vi "仪器控制1.vi"() -> ()   [LabVIEW 2018]
uses:
  <vilib>/Instr/_visa.llb/VISA Configure Serial Port (Instr).vi
panel:
  in  "截取采样时间下限":dbl
  in  "截取采样时间上限":dbl
  out "已循环周期数":i32
  in  "停止":bool
  out "x-y":u32
  out "停止按钮指示灯 2":bool
  out "大小":i32
  out "原始数据":dbl
  in  "偏差范围上限 2":dbl=5.0
  in  "偏差范围下限 2":dbl=5.0
  out "电流超出范围":bool=TRUE
  out "电流上限":dbl
  out "电流下限":dbl
  in  "截取下限时间 2":dbl
  in  "截取上限时间 2":dbl
  in  "截取下限时间":dbl=1.0
  in  "截取上限时间":dbl=10.0
  out "当前时间值":dbl
  out "波形图（采样频率不够无法完全拟合出曲线c）":dbl[](graph)
  out "子字符串之前 2":string
  out "双精度浮点数":dbl
  out "*(类型 *) &x":dbl
  out "实际输出电流":dbl
  out "子字符串之后":string
  out "匹配子字符串":string
  out "子字符串之前":string
  out "读取缓冲区":string
  out "运行按钮指示灯":bool
  in  "退出":bool
  in  "运行":bool
  in  "前段波形持续时间(s)":dbl=10.0
  in  "斜率决定因素":dbl=0.02
  in  "循环周期数":i32=30000
  out "第一周期近似波形图":dbl[](graph)
  in  "0安培电流保持时间":dbl=50.0
  in  "Time Resolution(s)":dbl=0.025
  in  "IR":dbl=20.0
  # "截取采样时间上限与斜率决定因素保持一致"
  # "配置"
  # "初始电流：50A 斜率决定因素：0.05\n初始电流：20A 斜率决定因素：0.02\n斜率决定因素值越小，越倾斜，但有过冲的风险越大\n总结：初始电流越大，斜率决定因素应越大"
  # "检测"
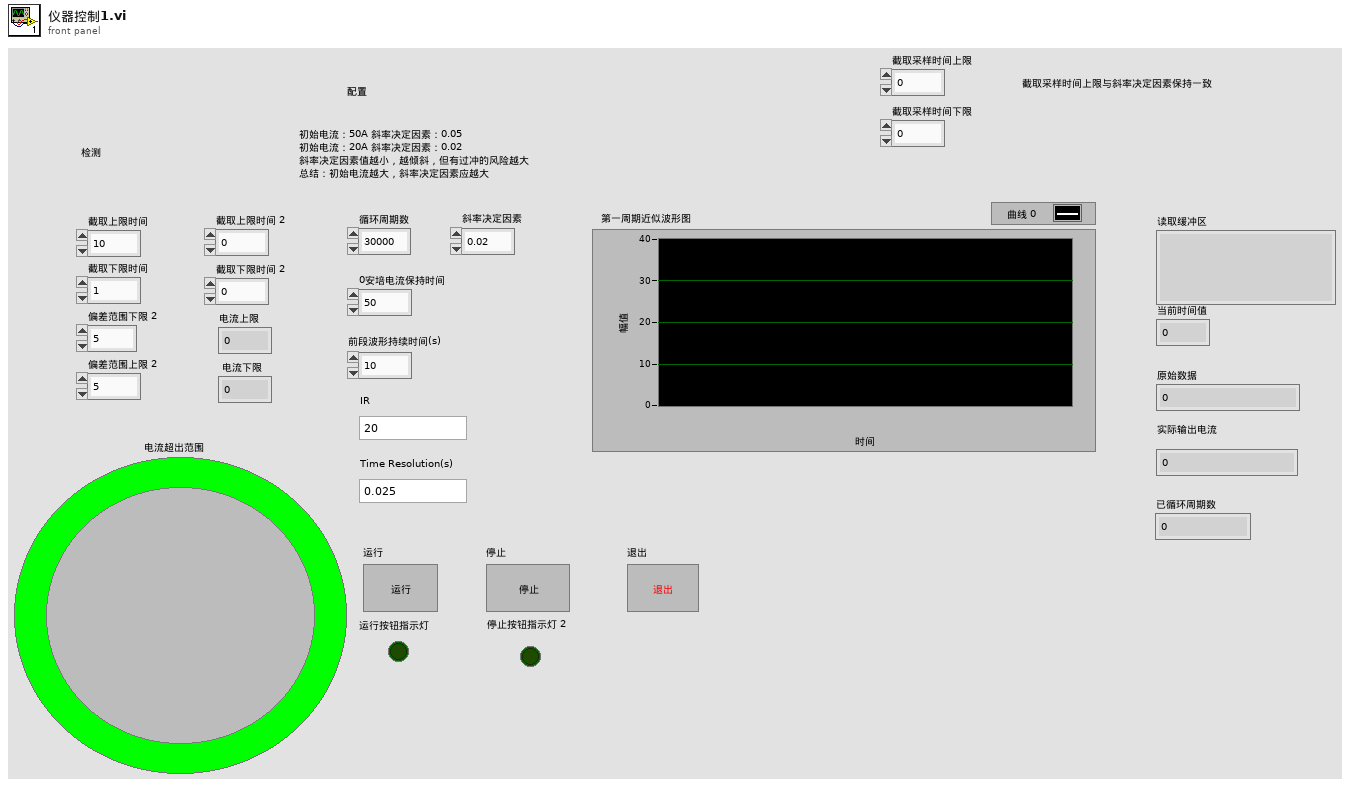
[diagram p1: front panel]
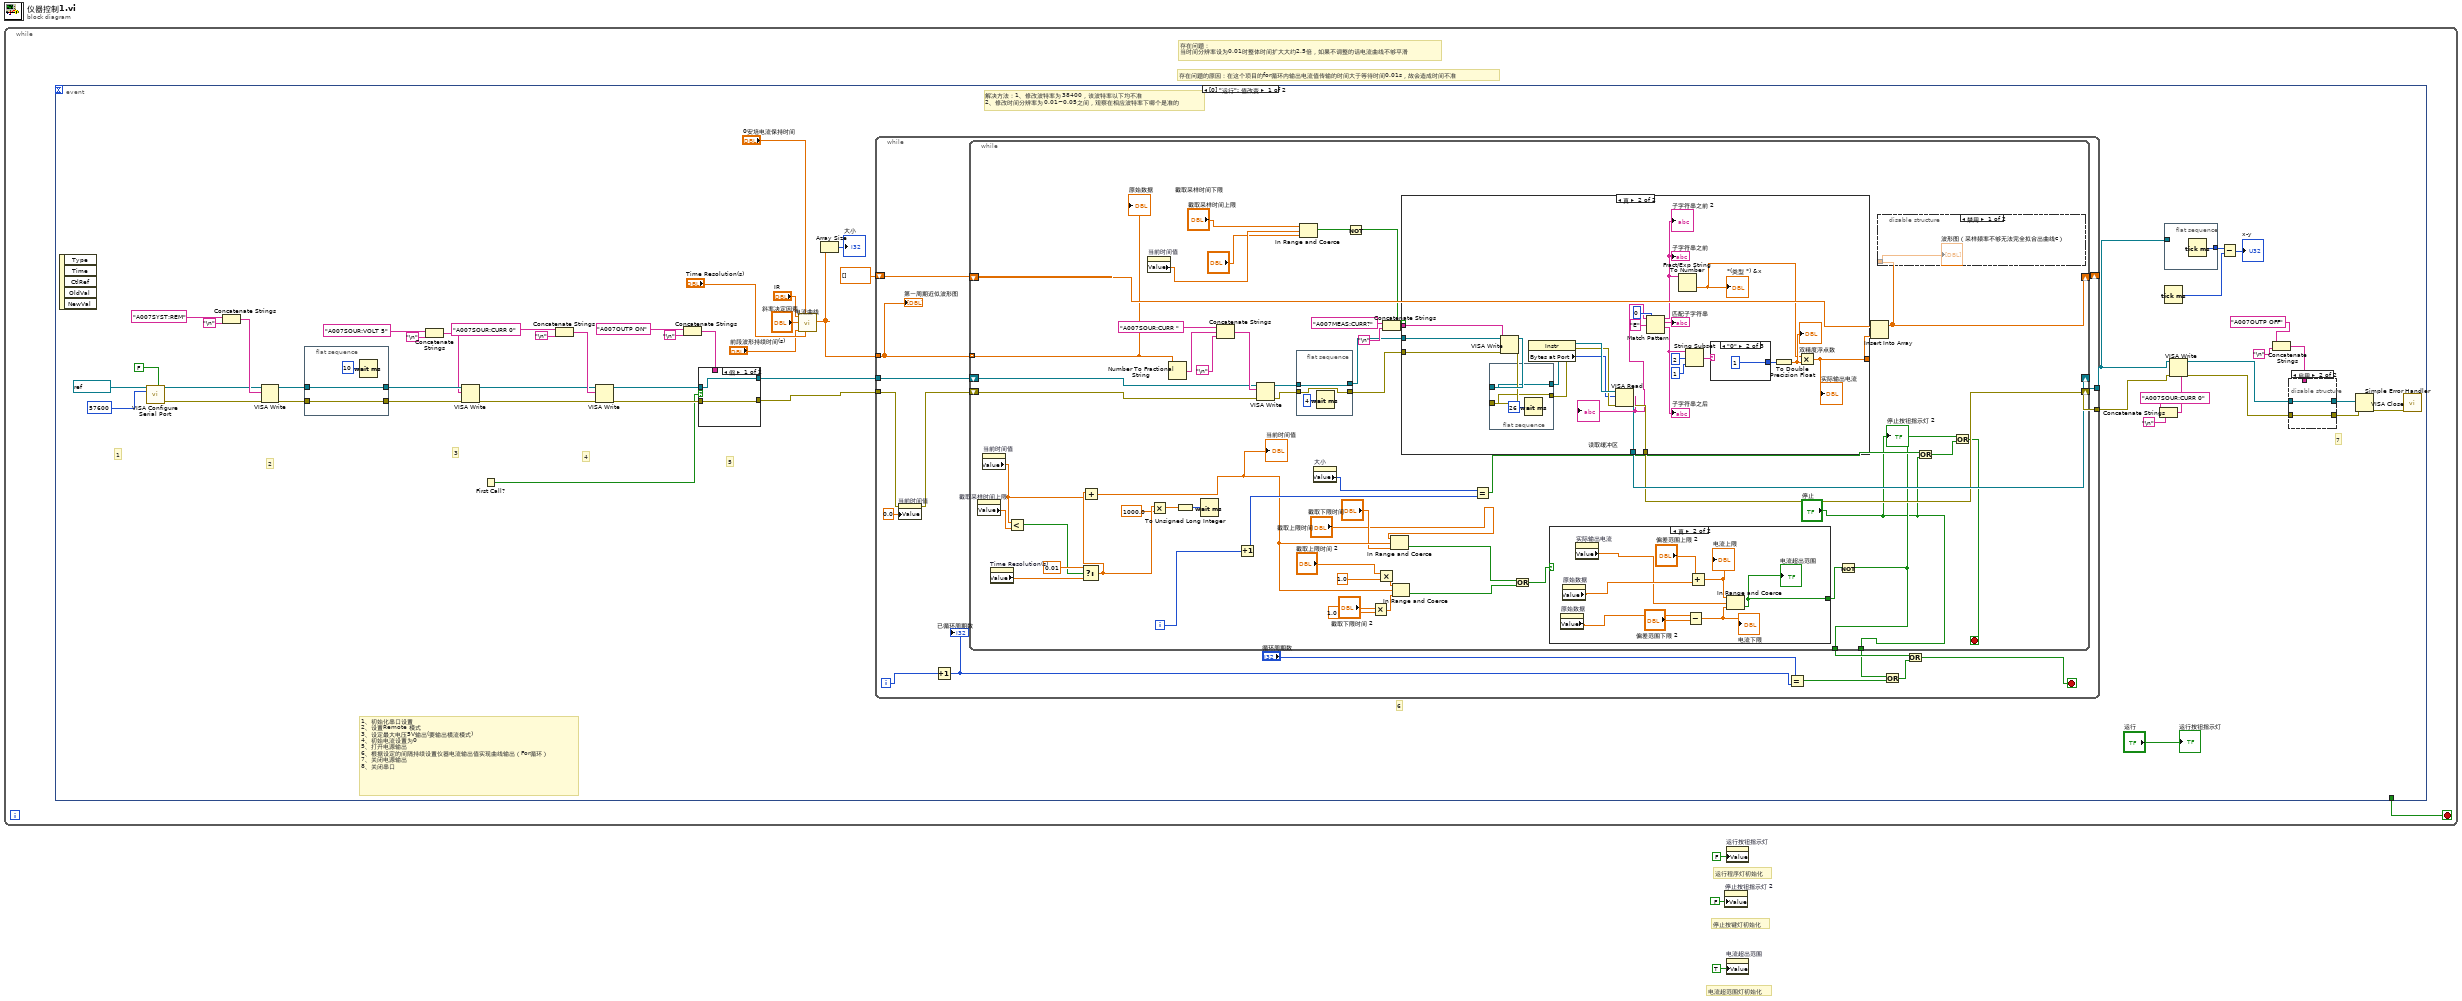
[diagram p0: block diagram]
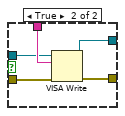
[diagram p2: hidden frame]
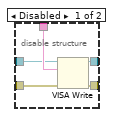
[diagram p3: hidden frame]
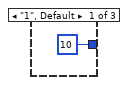
[diagram p5: hidden frame]
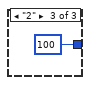
[diagram p6: hidden frame]
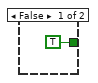
[diagram p8: hidden frame]
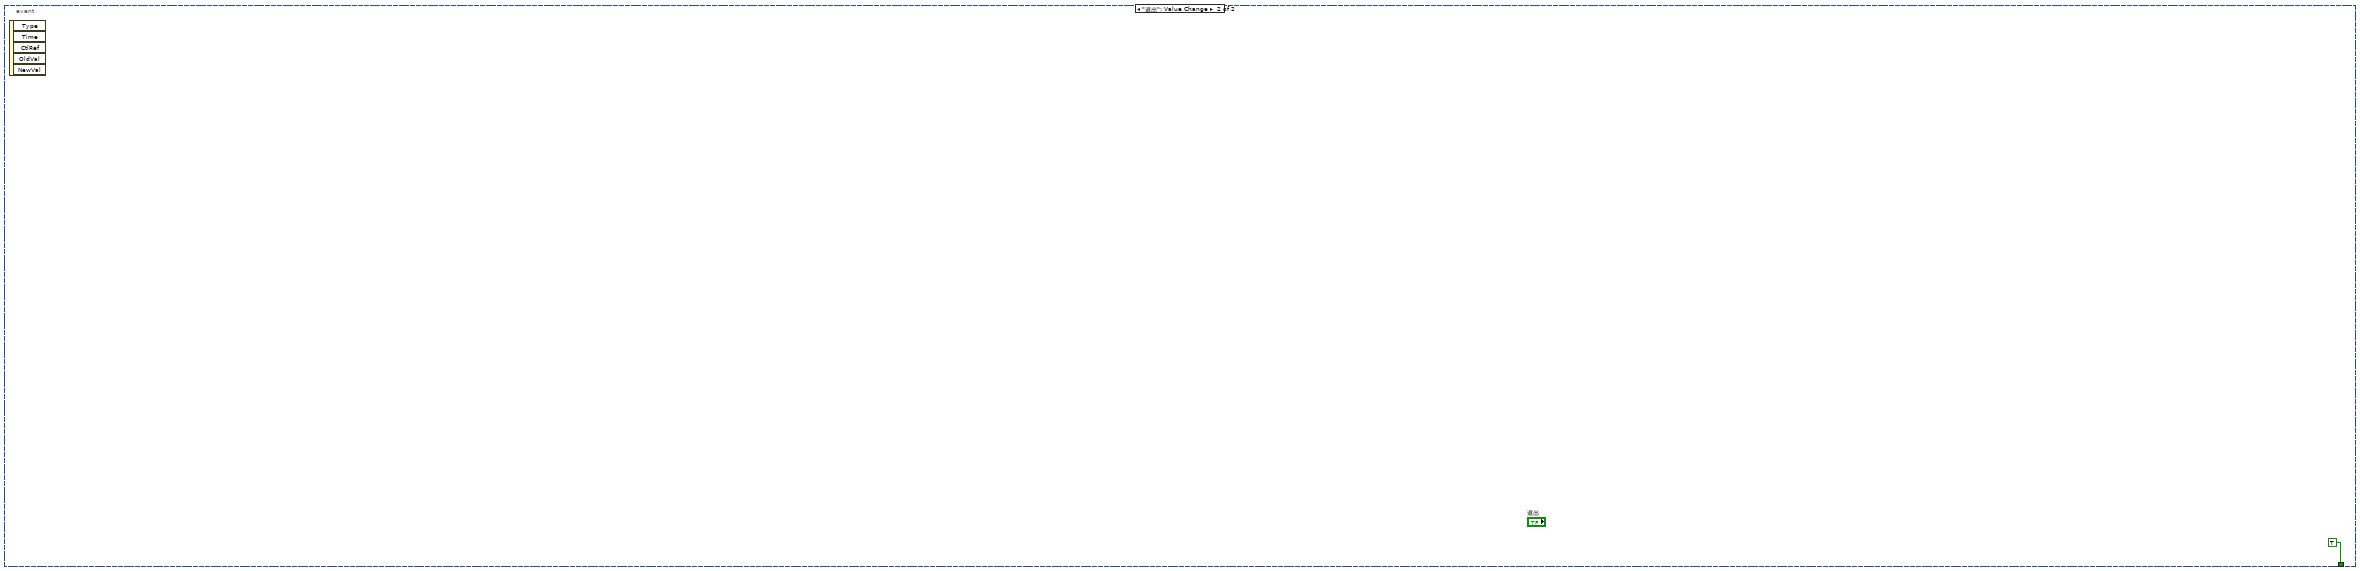
[diagram p9: hidden frame]
diagram:
  # "运行程序灯初始化"
  # "停止按键灯初始化"
  # "电流超范围灯初始化"
  n1 = while {
    stop <- w4 stop-if-true
    # "存在问题的原因：在这个项目的for循环内输出电流值传输的时间大于等待时间0.01s，故会造成时间不准"
    # "存在问题：\n当时间分辨率设为0.01时整体时间扩大大约2.5倍，如果不调整的话电流曲线不够平滑"
    n2 = event shown="[0] \"运行\": 值改变" {
      selector: _ -> [_ _]
      dyn-events: _ -> [_ _]
      timeout: _ -> [_ _]
      tunnel: [_ TRUE] -> w4
      event "运行": Value Change {
        # "6"
        # "解决方法：1、修改波特率为38400，该波特率以下均不准\n2、修改时间分辨率为0.01~0.05之间，观察在相应波特率下哪个是准的"
        # "7"
        # "5"
        # "4"
        # "3"
        # "2"
        # "1"
        # "1、初始化串口设置\n2、设置Remote 模式\n3、设定最大电压5V输出(要输出横流模式)\n4、初始电流设置为0\n5、打开电源输出\n6、根据设定的间隔持续设置仪器电流输出值实现曲线输出（For循环）\n7、关闭电源输出\n8、关闭串口"
        n3 = event-data() -> ()  [unwired: 1 in, 5 out]
        n4 = call-poly "VISA Configure Serial Port"("VISA resource name"=refnum<visa-resource-name> "COM3", "Enable Termination\nChar (T)"=FALSE ("Enable Termination\nChar (T)"), "baud rate (9600)"=u32 57600) -> ("VISA resource name out"=w49:refnum<visa-resource-name>, "error out"=w48:errorcluster)  [unwired: 11 in]
        n5 = Concatenate Strings("A007SYST:REM" ("字符串"), "\n") -> (w54:string)
        n6 = VISA Write(VISA resource name=w49, write buffer=w54, error in (no error)=w48) -> (VISA resource name out=w57:refnum<visa-resource-name>, error out=w56:errorcluster)  [unwired: 1 out]
        n7 = flat-sequence {
          tunnel: w57 -> [w191]
          tunnel: [w191] -> w46
          tunnel: w56 -> [w190]
          tunnel: [w190] -> w45
          frame #0 {
            n8 = Wait (ms)(milliseconds to wait=u32 10 ("等待时间（毫秒）")) -> ()  [unwired: 1 out]
          }
        }
        n9 = Concatenate Strings("A007SOUR:VOLT 5" ("字符串"), "\n") -> (w42:string)
        n10 = VISA Write(VISA resource name=w46, write buffer=w42, error in (no error)=w45) -> (VISA resource name out=w38:refnum<visa-resource-name>, error out=w37:errorcluster)  [unwired: 1 out]
        n11 = First Call?() -> (First Call?: T/F=w5:bool)
        n12 = Concatenate Strings("A007SOUR:CURR 0" ("字符串"), "\n") -> (w41:string)
        n13 = VISA Write(VISA resource name=w38, write buffer=w41, error in (no error)=w37) -> (VISA resource name out=w33:refnum<visa-resource-name>, error out=w32:errorcluster)  [unwired: 1 out]
        n14 = Concatenate Strings("A007OUTP ON" ("字符串"), "\n") -> (w34:string)
        n15 = case shown="假" w5 {
          tunnel: w34 -> [_ w64]
          tunnel: w33 -> [w59 w63]
          tunnel: w32 -> [w58 w62]
          tunnel: [w59 w61] -> w31
          tunnel: [w58 w60] -> w6
          frame False {
          }
          frame True {
            n16 = VISA Write(VISA resource name=w63, write buffer=w64, error in (no error)=w62) -> (VISA resource name out=w61:refnum<visa-resource-name>, error out=w60:errorcluster)  [unwired: 1 out]
          }
        }
        n17 = call "电流曲线.vi"("Time Resolution(s) 2"="Time Resolution(s)", "0安培电流保持时间"="0安培电流保持时间", "总持续时间(s)"="前段波形持续时间(s)", "x的第二个值决定斜率（建议0.02）"="斜率决定因素", "IR"="IR") -> ("输出电流值"=w18:dbl[])  [unwired: 6 in]
        n18 = Array Size(array=w18) -> (size(s)=→"大小":i32)
        n19 = while {
          tunnel: w31 -> [w89]
          tunnel: w6 -> [w73]
          tunnel: [w88] -> w7
          tunnel: [w87] -> w13
          tunnel: w18 -> [w86]
          shift-right: [w85] -> _
          shift-left: dbl[] [] -> [w84]
          i -> [w81]
          stop <- w77 stop-if-true
          n20 = property on="当前时间值" class="DigNum (严格)"(error in=w73, "Value"=0.0 ("当前时间值")) -> (error out=w74:errorcluster)  [unwired: 1 in, 1 out]
          n21 = Increment(x=w81) -> (x+1=w80:i32)
          "已循环周期数" <- w80
          n22 = while {
            tunnel: w86 -> [w114] mode=indexing
            shift-right: [w129] -> w87
            shift-left: w74 -> [w140]
            shift-right: [w130] -> w88
            shift-left: w89 -> [w141]
            shift-right: [w127] -> w85
            shift-left: w84 -> [w126]
            tunnel: [w108] -> w78
            tunnel: ["停止"] -> w76
            i -> [w116]
            stop <- w110 stop-if-true
            n23 = property on="截取采样时间上限" class="DigNum (严格)"() -> ("Value"=w90:dbl)  [unwired: 2 in, 2 out]
            n24 = property on="当前时间值" class="DigNum (严格)"() -> ("Value"=w98:dbl)  [unwired: 2 in, 2 out]
            n25 = property on="Time Resolution(s)" class="DigNum (严格)"() -> ("Value"=w103:dbl)  [unwired: 2 in, 2 out]
            n26 = Less?(x=w98, y=w90) -> (x < y?=w104:bool)
            n27 = Select(t=0.01 ("y"), s=w104, f=w103) -> (s? t:f=w102:dbl)
            n28 = Add(x=w102, y=w98) -> (x+y=w97:dbl)
            "当前时间值" <- w97
            n29 = property on="当前时间值" class="DigNum (严格)"() -> ("Value"=w96:dbl)  [unwired: 2 in, 2 out]
            n30 = Multiply(x=w102, y=1000.0) -> (x*y=w99:dbl)
            n31 = Number To Fractional String(number=w114) -> (F-format string=w138:string)  [unwired: 3 in]
            n32 = To Unsigned Long Integer(number=w99) -> (unsigned 32bit integer=w100:u32)
            n33 = Wait (ms)(milliseconds to wait=w100) -> ()  [unwired: 1 out]
            n34 = Concatenate Strings("A007SOUR:CURR " ("字符串"), w138, "\n") -> (w142:string)
            n35 = Increment(x=w116) -> (x+1=w125:i32)
            n36 = VISA Write(VISA resource name=w141, write buffer=w142, error in (no error)=w140) -> (VISA resource name out=w136:refnum<visa-resource-name>, error out=w137:errorcluster)  [unwired: 1 out]
            n37 = flat-sequence {
              tunnel: w137 -> [w187]
              tunnel: w136 -> [w188]
              tunnel: [w188] -> w132
              tunnel: [w187] -> w131
              frame #0 {
                n38 = Wait (ms)(milliseconds to wait=u32 4 ("等待时间（毫秒）")) -> ()  [unwired: 1 out]
              }
            }
            n39 = In Range and Coerce(upper limit="截取采样时间上限", x=w96, lower limit="截取采样时间下限") -> (In Range?=w106:bool)  [unwired: 1 out]
            n40 = property on="大小" class="DigNum (严格)"() -> ("Value"=w113:i32)  [unwired: 2 in, 2 out]
            n41 = Not(x=w106) -> (.not. x?=w95:bool)
            n42 = Multiply(x="截取下限时间 2", y=1.0) -> (x*y=w120:dbl)
            n43 = Multiply(x="截取上限时间 2", y=1.0) -> (x*y=w117:dbl)
            n44 = Concatenate Strings("A007MEAS:CURR?" ("字符串"), "\n") -> (w133:string)
            n45 = In Range and Coerce(upper limit="截取上限时间", x=w97, lower limit="截取下限时间") -> (In Range?=w123:bool)  [unwired: 1 out]
            n46 = In Range and Coerce(upper limit=w117, x=w97, lower limit=w120) -> (In Range?=w124:bool)  [unwired: 1 out]
            n47 = case shown="真" w95 {
              tunnel: w133 -> [_ w170]
              tunnel: w132 -> [w145 w169]
              tunnel: w131 -> [w144 w168]
              tunnel: [w145 w161] -> w130
              tunnel: [w144 w160] -> w129
              tunnel: [_ w149] -> w128
              frame False {
              }
              frame True {
                n48 = flat-sequence {
                  tunnel: w167 -> [w175]
                  tunnel: w166 -> [w174]
                  tunnel: [w175] -> w165
                  tunnel: [w174] -> w164
                  frame #0 {
                    n49 = Wait (ms)(milliseconds to wait=u32 26 ("等待时间（毫秒）")) -> ()  [unwired: 1 out]
                  }
                }
                n50 = VISA Write(VISA resource name=w169, write buffer=w170, error in (no error)=w168) -> (VISA resource name out=w167:refnum<visa-resource-name>, error out=w166:errorcluster)  [unwired: 1 out]
                n51 = property class="Instr"(reference=w165, error in=w164) -> (reference out=w163:refnum<visa-resource-name>, error out=w162:errorcluster, "Bytes at Port"=w159:u32)
                n52 = VISA Read(VISA resource name=w163, byte count=w159, error in (no error)=w162) -> (VISA resource name out=w161:refnum<visa-resource-name>, read buffer=w146:string, error out=w160:errorcluster)  [unwired: 1 out]
                "读取缓冲区" <- w146
                n53 = Match Pattern(string=w146, regular expression="E" ("正则表达式"), offset (0)=0 ("偏移量(0)")) -> (before substring=w151:string, match substring=→"匹配子字符串":string, after substring=w157:string)  [unwired: 1 out]
                "子字符串之前" <- w151
                "子字符串之后" <- w157
                "子字符串之前 2" <- w151
                n54 = Fract/Exp String To Number(string=w151) -> (number=w150:dbl)  [unwired: 3 in, 1 out]
                "*(类型 *) &x" <- w150
                n55 = String Subset(string=w157, offset (0)=2 ("偏移量(0)"), length (rest)=1 ("长度（剩余）")) -> (substring=w154:string)
                n56 = case shown="\"0\"" w154 {
                  tunnel: [10 1 100] -> w152
                  frame "1", Default {
                  }
                  frame "0" {
                  }
                  frame "2" {
                  }
                }
                n57 = To Double Precision Float(number=w152) -> (double precision float=w153:dbl)
                "双精度浮点数" <- w153
                n58 = Multiply(x=w150, y=w153) -> (x*y=w149:dbl)
                "实际输出电流" <- w149
              }
            }
            n59 = Equal?(x=w113, y=w125) -> (x = y?=w111:bool)
            n60 = Or(x=w123, y=w124) -> (x .or. y?=w115:bool)
            n61 = case shown="真" w115 {
              tunnel: [TRUE w182] -> w109
              frame False {
              }
              frame True {
                n62 = property on="原始数据" class="DigNum (严格)"() -> ("Value"=w180:dbl)  [unwired: 2 in, 2 out]
                n63 = property on="原始数据" class="DigNum (严格)"() -> ("Value"=w181:dbl)  [unwired: 2 in, 2 out]
                n64 = property on="实际输出电流" class="DigNum (严格)"() -> ("Value"=w179:dbl)  [unwired: 2 in, 2 out]
                n65 = Subtract(x=w180, y="偏差范围下限 2") -> (x-y=w184:dbl)
                "电流下限" <- w184
                n66 = Add(x="偏差范围上限 2", y=w181) -> (x+y=w186:dbl)
                "电流上限" <- w186
                n67 = In Range and Coerce(upper limit=w186, x=w179, lower limit=w184) -> (In Range?=w182:bool)  [unwired: 1 out]
                "电流超出范围" <- w182
              }
            }
            n68 = Not(x=w109) -> (.not. x?=w108:bool)
            n69 = Insert Into Array(array=w126, new element=w128) -> (w127:dbl[])  [unwired: 1 in]
            n70 = disable-structure shown="禁用" {
              disable-tunnel: w127 -> [w177 _]
              frame Disabled {
                "波形图（采样频率不够无法完全拟合出曲线c）" <- w177
              }
              frame Enabled {
              }
            }
            n71 = Or(x=w111, y="停止") -> (x .or. y?=w112:bool)
            n72 = Or(x=w108, y=w112) -> (x .or. y?=w110:bool)
            "原始数据" <- w114
            "停止按钮指示灯 2" <- "停止"
          }
          n73 = Equal?(x="循环周期数", y=w80) -> (x = y?=w83:bool)
          n74 = Or(x=w76, y=w83) -> (x .or. y?=w82:bool)
          n75 = Or(x=w78, y=w82) -> (x .or. y?=w77:bool)
          "第一周期近似波形图" <- w86
        }
        n76 = Concatenate Strings("A007SOUR:CURR 0", "\n") -> (w16:string)
        n77 = flat-sequence {
          tunnel: [w72] -> w10
          tunnel: w7 -> [_]
          frame #0 {
            n78 = Tick Count (ms)() -> (millisecond timer value=w72:u32)
          }
        }
        n79 = Tick Count (ms)() -> (millisecond timer value=w9:u32)
        n80 = VISA Write(VISA resource name=w7, write buffer=w16, error in (no error)=w13) -> (VISA resource name out=w12:refnum<visa-resource-name>, error out=w11:errorcluster)  [unwired: 1 out]
        n81 = Subtract(x=w10, y=w9) -> (x-y=→"x-y":u32)
        n82 = Concatenate Strings("A007OUTP OFF" ("字符串"), "\n") -> (w30:string)
        n83 = disable-structure shown="启用" {
          disable-tunnel: w30 -> [w69 _]
          disable-tunnel: [w68 w71] -> w27
          disable-tunnel: [w67 w70] -> w26
          disable-tunnel: w12 -> [w66 w71]
          disable-tunnel: w11 -> [w65 w70]
          frame Disabled {
            n84 = VISA Write(VISA resource name=w66, write buffer=w69, error in (no error)=w65) -> (VISA resource name out=w68:refnum<visa-resource-name>, error out=w67:errorcluster)  [unwired: 1 out]
          }
          frame Enabled {
          }
        }
        n85 = VISA Close(VISA resource name=w27, error in (no error)=w26) -> (error out=w52:errorcluster)
        n86 = call <vilib>:"Simple Error Handler.vi"("error in (no error)"=w52) -> ()  [unwired: 4 in, 5 out]
        "运行按钮指示灯" <- "运行"
      }
      event "退出": Value Change {
        n87 = event-data() -> ()  [unwired: 1 in, 5 out]
      }
    }
  }
  n88 = property on="停止按钮指示灯 2" class="Bool (严格)"("Value"=FALSE ("停止按钮指示灯 2")) -> ()  [unwired: 2 in, 2 out]
  n89 = property on="运行按钮指示灯" class="Bool (严格)"("Value"=FALSE ("运行按钮指示灯")) -> ()  [unwired: 2 in, 2 out]
  n90 = property on="电流超出范围" class="Bool (严格)"("Value"=TRUE ("电流超出范围")) -> ()  [unwired: 2 in, 2 out]
